vi "WSVCAP SHL Host TL I2C Write - Single Device.vi"(0 "Sub Address [U8]":u8=20 format="%.0x", 5 "Data Out [U8]":u8=20 format="%.0x", 11 "error in":errorcluster, 12 "DUT":T1, 13 "Device":T2, 14 "Log (T)":bool=TRUE) -> (15 "error out":errorcluster)   [LabVIEW 2012]
uses:
  Type Defs/WSVCAP SHL I2C Device Enum.ctl
  Type Defs/WSVCAP SHL DUT Number Enum.ctl
panel:
  out "C3 Data Out [U8]":u8[](array[numeric]) format="%.0x"
  out "Socket Mask Set [U64]":u64[](array[numeric]) format="%012x"
  out "C2 Data Out [U8]":u8[](array[numeric]) format="%.0x"
  out "C1 Data Out [U8]":u8[](array[numeric]) format="%.0x"
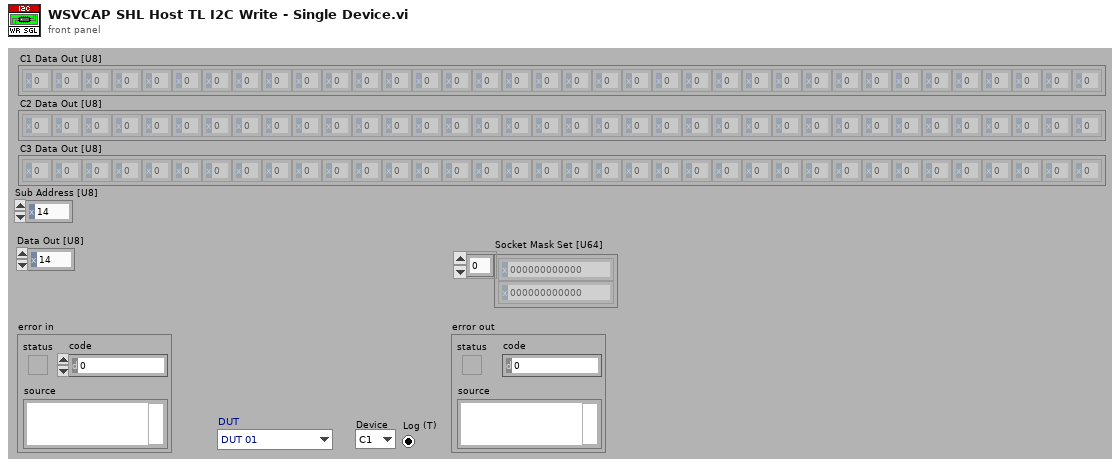
[diagram p1: front panel]
types:
  T1 = typedef "WSVCAP SHL DUT Number Enum.ctl" = enum16{"DUT 01", "DUT 02", "DUT 03", "DUT 04", "DUT 05", "DUT 06", "DUT 07", "DUT 08", "DUT 09", "DUT 10", "DUT 11", "DUT 12", "DUT 13", "DUT 14", "DUT 15", "DUT 16", "DUT 17", "DUT 18", "DUT 19", "DUT 20", "DUT 21", "DUT 22", "DUT 23", "DUT 24", "DUT 25", "DUT 26", "DUT 27", "DUT 28", "DUT 29", "DUT 30", "DUT 31", "DUT 32", "DUT 33", "DUT 34", "DUT 35", "DUT 36"}
  T2 = typedef "WSVCAP SHL I2C Device Enum.ctl" = enum16{"C1", "C2", "C3"}
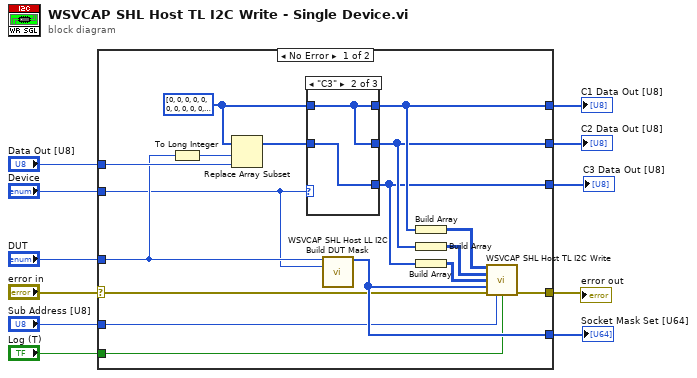
[diagram p0: block diagram]
diagram:
  n1 = case shown="No Error" "error in" {
    selector: "error in" -> [w17 w35]
    tunnel: [w28 w35] -> w11
    tunnel: "Sub Address [U8]" -> [w14 _]
    tunnel: "Data Out [U8]" -> [w27 _]
    tunnel: "Device" -> [w16 _]
    tunnel: [w21 _] -> w6
    tunnel: [w22 _] -> w5
    tunnel: "DUT" -> [w23 _]
    tunnel: [w18 _] -> w3
    tunnel: "Log (T)" -> [w15 _]
    tunnel: [w13 _] -> w1
    frame No Error {
      w25 = u8[] [0, 0, 0, 0, 0, 0, 0, 0, 0, 0, 0, 0, 0, 0, 0, 0, 0, 0, 0, 0, 0, 0, 0, 0, 0, 0, 0, 0, 0, 0, 0, 0, 0, 0, 0, 0] ("SPI Data Out")
      n2 = To Long Integer(number=w23) -> (32bit integer=w26:i32)
      n3 = Replace Array Subset(array=w25, new element=w27, index=w26) -> (w24:u8[])
      n4 = case shown="\"C3\"" w16 {
        tunnel: [w29 w31 w34] -> w22
        tunnel: w25 -> [w29 w31 w33]
        tunnel: [w30 w31 w33] -> w21
        tunnel: w24 -> [w30 w32 w34]
        tunnel: [w29 w32 w33] -> w13
        frame "C2" {
        }
        frame "C3" {
        }
        frame "C1" {
        }
      }
      n5 = call "WSVCAP SHL Host LL I2C Build DUT Mask.vi"("DUT"=w23, "Device"=w16) -> ("Socket Mask Set [U64]"=w18:u64[])  [unwired: 12 in, 1 out]
      n6 = Build Array(w22) -> (w20:u8[][])
      n7 = Build Array(w21) -> (w19:u8[][])
      n8 = Build Array(w13) -> (w12:u8[][])
      n9 = call "WSVCAP SHL Host TL I2C Write.vi"("C1 Data Out"=w20, "C2 Data Out"=w19, "C3 Data Out"=w12, "Socket Mask Set [U64]"=w18, "error in"=w17, "Sub Address"=w14, "Log (T)"=w15) -> ("error out"=w28:errorcluster)  [unwired: 8 in]
    }
    frame Error {
    }
  }
  "error out" <- w11
  "C1 Data Out [U8]" <- w5
  "C2 Data Out [U8]" <- w6
  "Socket Mask Set [U64]" <- w3
  "C3 Data Out [U8]" <- w1
